vi "Configure Channel (Volt Scale).vi"(0 "VISA resource name":refnum<visa-resource-name>, 1 "Scaling":T2={"Floating Point Position (2)"=2, "Lower Scaling (0)"=0.0, "Upper Scaling (10000)"=100.0, "Unit Character (\"\")"=""} {"Upper Scaling (10000)" format="%_6g"; "Lower Scaling (0)" format="%_6g"; "Floating Point Position (2)" min=0 max=5 step=1}, 5 "Channel (0001)":string="0001", 7 "Enable Channel (True)":bool=TRUE, 9 "Range And Span":T1={"Volt Range (4 : 2V)"=4, "Enable Span (False)"=FALSE, "Lower Span (2.0000)"=-2.0, "Upper Span (2.0000)"=2.0, "Bias (0)"=0.0} {"Upper Span (2.0000)" min=-99999.0 max=99999.0 step=1.0 format="%_5g"; "Lower Span (2.0000)" min=-99999.0 max=99999.0 step=1.0 format="%_5g"; "Volt Range (4 : 2V)" items=["20mV", "60mV", "200mV", "1V", "2V", "6V", "20V", "50V"]}, 11 "error in (no error)":errorcluster) -> (4 "VISA resource name out":refnum<visa-resource-name>, 6 "Channel":string, 15 "error out":errorcluster)   [LabVIEW 2020, in "Yokogawa GX Series.lvlib"]
doc: "Sets the input range as voltage.\n\nCommand: SRangeAI"
uses:
  <instrlib>/Yokogawa GX Series/Yokogawa GX Series.lvlib
  <instrlib>/Yokogawa GX Series/Private/Volt Range.vi
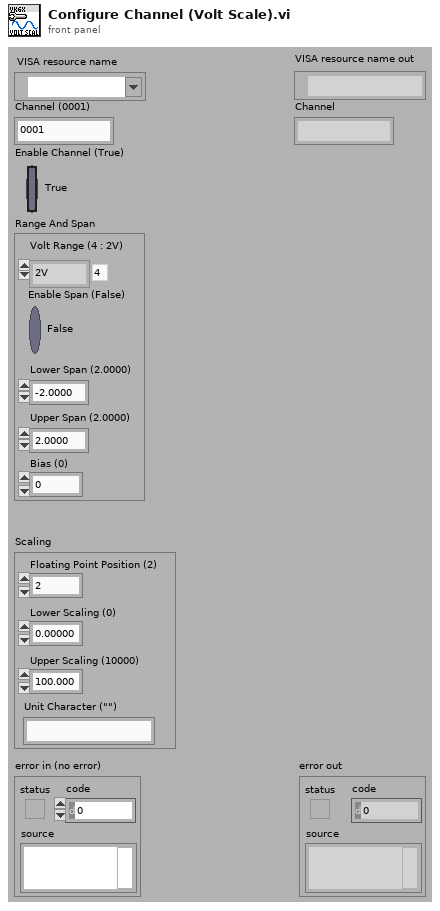
[diagram p1: front panel]
types:
  T1 = cluster{"Volt Range (4 : 2V)":i32, "Enable Span (False)":bool, "Lower Span (2.0000)":dbl, "Upper Span (2.0000)":dbl, "Bias (0)":dbl}
  T2 = cluster{"Floating Point Position (2)":i32, "Lower Scaling (0)":dbl, "Upper Scaling (10000)":dbl, "Unit Character (\"\")":string}
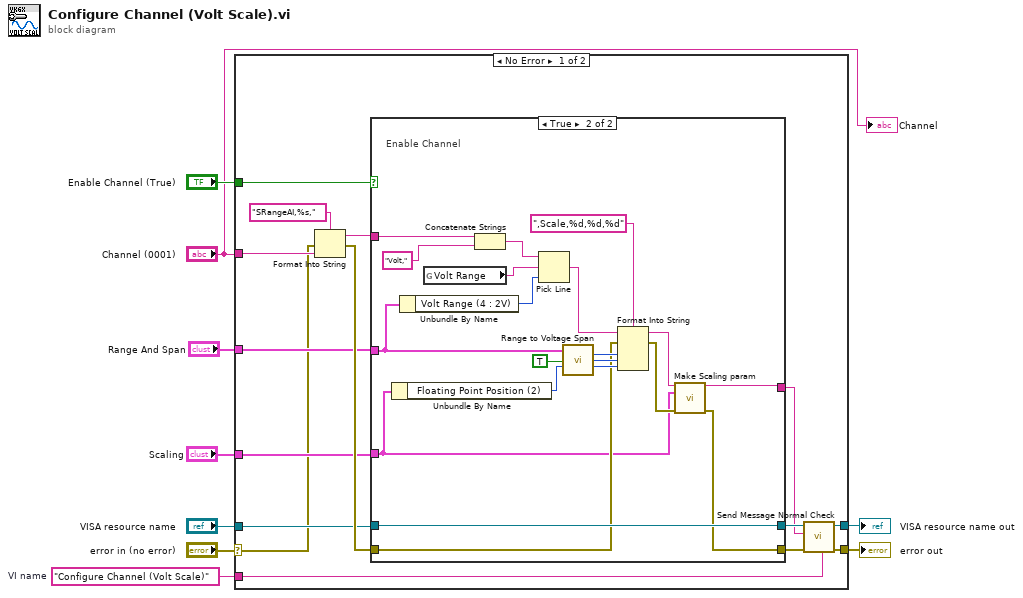
[diagram p0: block diagram]
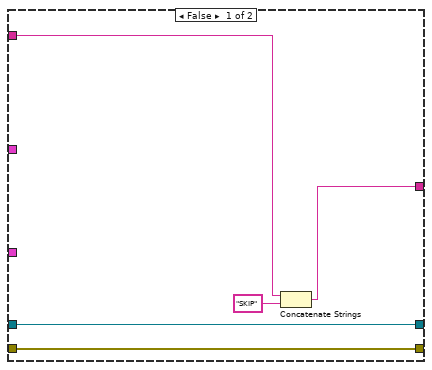
[diagram p2: hidden frame]
diagram:
  w5 = "Configure Channel (Volt Scale)"  # VI name
  n1 = case shown="No Error" "error in (no error)" {
    selector: "error in (no error)" -> [w10 w50]
    tunnel: "VISA resource name" -> [w21 w51]
    tunnel: "Scaling" -> [w20 _]
    tunnel: [w17 w51] -> w7
    tunnel: [w16 w50] -> w6
    tunnel: w5 -> [w14 _]
    tunnel: "Range And Span" -> [w13 _]
    tunnel: "Enable Channel (True)" -> [w12 _]
    tunnel: "Channel (0001)" -> [w11 _]
    frame No Error {
      n2 = Format Into String(format string="SRangeAI,%s,", error in=w10, w11) -> (resulting string=w22:string, error out=w23:errorcluster)  [unwired: 1 in]
      n3 = case shown="True" w12 {
        tunnel: w23 -> [w26 w40]
        tunnel: [w26 w36] -> w18
        tunnel: w22 -> [w28 w47]
        tunnel: [w29 w34] -> w15
        tunnel: w21 -> [w25 w41]
        tunnel: [w25 w41] -> w19
        tunnel: w20 -> [_ w32]
        tunnel: w13 -> [_ w39]
        frame False {
          n4 = Concatenate Strings(w28, "SKIP") -> (w29:string)
        }
        frame True {
          # "Enable Channel"
          n5 = Unbundle By Name(w32) -> ("Floating Point Position (2)"=w35:i32)
          n6 = Unbundle By Name(w39) -> ("Volt Range (4 : 2V)"=w45:i32)
          n7 = global read "Volt Range.vi" "Volt Range"() -> (w30:string)
          n8 = Concatenate Strings(w47, "Volt,") -> (w46:string)
          n9 = Pick Line(string ("")=w46, multi-line string=w30, line index=w45) -> (output string=w48:string)
          n10 = call <instrlib>:"Range to Voltage Span.vi"("Range And Span"=w39, "Scaling? (False)"=TRUE, "Floating Point Position (2)"=w35) -> ("Lower Span"=w44:i32, "Upper Span"=w43:i32, "Bias"=w42:i32)  [unwired: 5 in, 5 out]
          n11 = Format Into String(format string=",Scale,%d,%d,%d", initial string=w48, error in=w40, w44, w43, w42) -> (resulting string=w33:string, error out=w37:errorcluster)
          n12 = call <instrlib>:"Make Scaling param.vi"("String (\"\")"=w33, "Scaling"=w32, "error in (no error)"=w37) -> ("String After"=w34:string, "error out"=w36:errorcluster)  [unwired: 11 in]
        }
      }
      n13 = call <instrlib>:"Send Message Normal Check.vi"("Source (\"\")"=w14, "error in (no error)"=w18, "Send Message (\"\")"=w15, "VISA resource name"=w19) -> ("error out"=w16:errorcluster, "VISA resource name out"=w17:refnum<visa-resource-name>)  [unwired: 2 in, 4 out]
    }
    frame Error {
    }
  }
  "error out" <- w6
  "VISA resource name out" <- w7
  "Channel" <- "Channel (0001)"
